vi "Create Connection.vi"(8 "error in (no error)":errorcluster, 11 "TCP Server in":refnum<class "TCP Server.lvclass">) -> (0 "error out":errorcluster, 2 "Connection":refnum<class "IConnection.lvclass">, 3 "TCP Server out":refnum<class "TCP Server.lvclass">)   [LabVIEW 2017, in "TCP Interface.lvlib" / "TCP Server.lvclass"]
uses:
  <vilib>/gpm_packages/@cs/Network-sink/Source/TCP Interface/TCP Server/TCP Server.lvclass
  <vilib>/gpm_packages/@cs/Network-sink/Source/Network Interface/IConnection/IConnection.lvclass
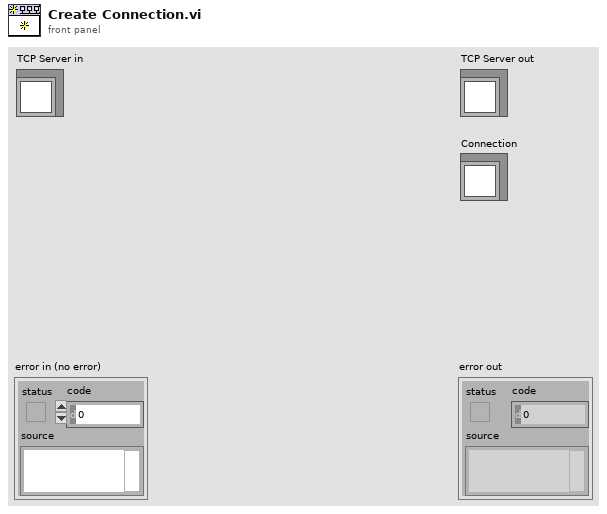
[diagram p1: front panel]
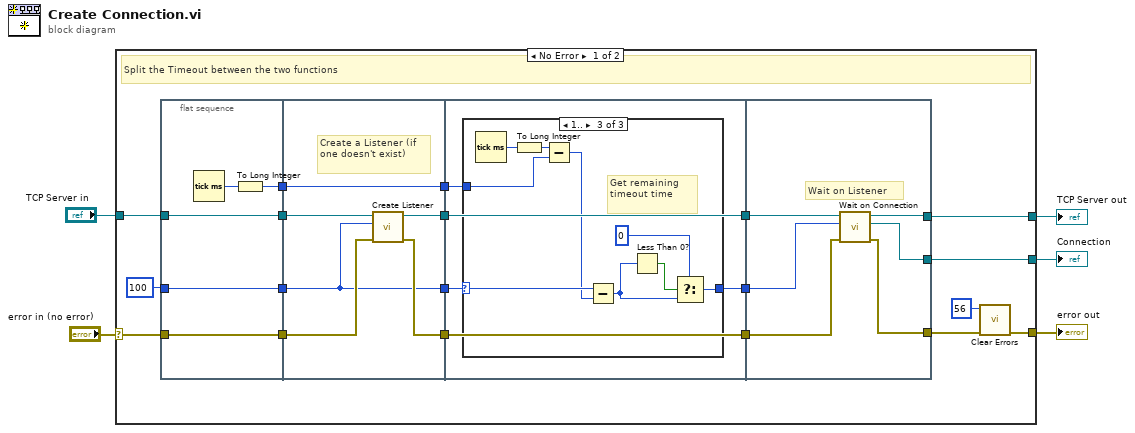
[diagram p0: block diagram]
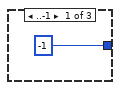
[diagram p2: hidden frame]
diagram:
  n1 = case shown="No Error" "error in (no error)" {
    selector: "error in (no error)" -> [w23 w58]
    tunnel: "TCP Server in" -> [w24 w59]
    tunnel: [w22 w59] -> w3
    tunnel: [w19 w58] -> w2
    tunnel: [w20 _] -> w1
    frame No Error {
      # "Split the Timeout between the two functions"
      n2 = flat-sequence {
        tunnel: 100 ("Timeout (25000 ms)") -> [w28]
        tunnel: w24 -> [w29]
        tunnel: [w29] -> w17
        tunnel: [w28] -> w16
        tunnel: [w25] -> w15
        tunnel: [w26] -> w14
        tunnel: w23 -> [w26]
        tunnel: w17 -> [w35]
        tunnel: w16 -> [w30]
        tunnel: w15 -> [w31]
        tunnel: w14 -> [w34]
        tunnel: [w33] -> w13
        tunnel: [w32] -> w12
        tunnel: [w31] -> w11
        tunnel: [w30] -> w10
        tunnel: w13 -> [w40]
        tunnel: w12 -> [w39]
        tunnel: w11 -> [w38]
        tunnel: [w40] -> w9
        tunnel: [w39] -> w8
        tunnel: w10 -> [w37]
        tunnel: [w36] -> w7
        tunnel: [w54] -> w21
        tunnel: w9 -> [w57]
        tunnel: w8 -> [w55]
        tunnel: [w56] -> w22
        tunnel: w7 -> [w53]
        tunnel: [w52] -> w20
        frame #0 {
          n3 = Tick Count (ms)() -> (millisecond timer value=w27:u32)
          n4 = To Long Integer(number=w27) -> (32bit integer=w25:i32)
        }
        frame #1 {
          # "Create a Listener (if one doesn't exist)"
          n5 = call <vilib>:"Create Listener.vi"("error in (no error)"=w34, "Timeout ms (25000)"=w30, "TCP Server in"=w35) -> ("error out"=w32:errorcluster, "TCP Server out"=w33:refnum<class "TCP Server.lvclass">)  [unwired: 7 in]
        }
        frame #2 {
          n6 = case shown="1.." w37 {
            selector: w37 -> [_ w42 w49]
            tunnel: w38 -> [_ _ w50]
            tunnel: [-1 ("t") w42 w44] -> w36
            frame ..-1 {
            }
            frame 0 {
            }
            frame 1.. {
              # "Get remaining timeout time"
              n7 = Tick Count (ms)() -> (millisecond timer value=w51:u32)
              n8 = To Long Integer(number=w51) -> (32bit integer=w47:i32)
              n9 = Subtract(x=w47, y=w50) -> (x-y=w48:i32)
              n10 = Subtract(x=w49, y=w48) -> (x-y=w45:i32)
              n11 = Less Than 0?(x=w45) -> (x < 0?=w46:bool)
              n12 = Select(t=0, s=w46, f=w45) -> (s? t:f=w44:i32)
            }
          }
        }
        frame #3 {
          # "Wait on Listener"
          n13 = call <vilib>:"Wait on Connection.vi"("error in (no error)"=w55, "Timeout (25000 ms)"=w53, "TCP Server in"=w57) -> ("error out"=w54:errorcluster, "Connection"=w52:refnum<class "IConnection.lvclass">, "TCP Server out"=w56:refnum<class "TCP Server.lvclass">)  [unwired: 6 in]
        }
      }
      n14 = call <vilib>:"Clear Errors.vi"("error in (no error)"=w21, "specific error code to clear (0: all)"=56) -> ("error out"=w19:errorcluster)  [unwired: 4 in, 1 out]
    }
    frame Error {
    }
  }
  "error out" <- w2
  "TCP Server out" <- w3
  "Connection" <- w1
